vi "Get Font.vi"(8 "error in":errorcluster, 11 "Cell in":refnum<class "Cell.lvclass">) -> (0 "error out":errorcluster, 2 "Font out":refnum<class "Font.lvclass">, 3 "Cell out":refnum<class "Cell.lvclass">)   [LabVIEW 2023, in "SourceGrid.lvlib" / "Cell.lvclass"]
uses:
  Cell.lvclass
  Font/Font.lvclass
  Cell.lvclass/Cell.ctl
  D:/git/Sourcegrid-LabVIEW/dll/SourceGrid.dll
  dll/SourceGrid.dll
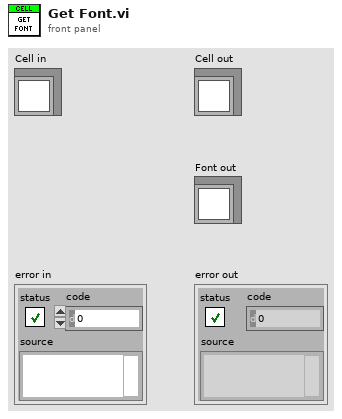
[diagram p1: front panel]
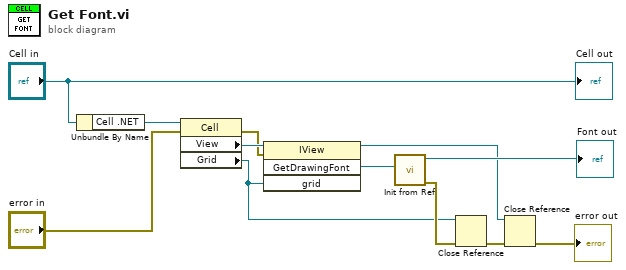
[diagram p0: block diagram]
diagram:
  n1 = Unbundle By Name("Cell in") -> ("Cell .NET"=w11:refnum<k24>)
  n2 = property class="Cell"(reference=w11, error in="error in") -> (error out=w4:errorcluster, "View"=w10:refnum<k24>, "Grid"=w1:refnum<k24>)  [unwired: 1 out]
  n3 = invoke class="IView" method="GetDrawingFont"(reference=w10, error in=w4, "grid"=w1) -> (reference out=w5:refnum<k24>, "GetDrawingFont"=w3:refnum<k24>)  [unwired: 1 in, 2 out]
  n4 = call "Init from Ref.vi"("Font"=w3) -> ("error out"=w7:errorcluster, "Font out"=→"Font out":refnum<class "Font.lvclass">)  [unwired: 9 in]
  n5 = Close Reference(reference=w1, error in (no error)=w7) -> (error out=w2:errorcluster)
  n6 = Close Reference(reference=w5, error in (no error)=w2) -> (error out=→"error out":errorcluster)
  "Cell out" <- "Cell in"
